vi "SET AO.vi"(8 "error in (no error)":errorcluster, 10 "Cluster SET AO":T1) -> (0 "error out":errorcluster)   [LabVIEW 2019]
uses:
  SET ARRAY AO.ctl
  SET SINGLE AO.ctl
  AO List.ctl
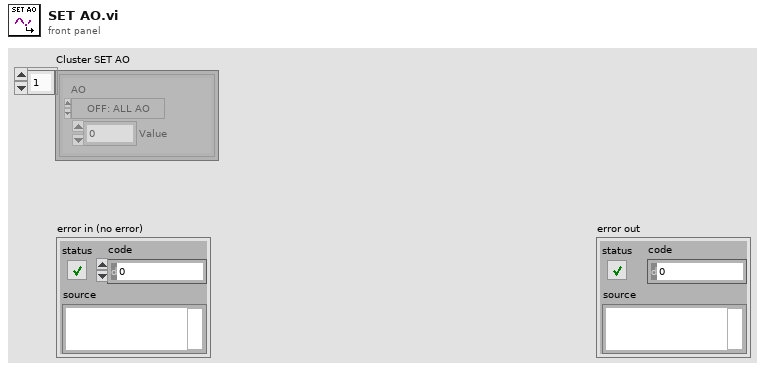
[diagram p1: front panel]
types:
  T1 = typedef "SET ARRAY AO.ctl" = T2[]
  T2 = typedef "SET SINGLE AO.ctl" = cluster{"AO":T3, "Value":dbl}
  T3 = typedef "AO List.ctl" = enum16{"OFF: ALL AO", "RIF VEL FRENO 1", "RIF VEL FRENO 2", "RIF VEL FRENO 3", "RIF COPPIA FRENO", "RIF COPPIA FRENO 1", "RIF COPPIA FRENO 2", "RIF COPPIA FRENO 3", "RIF CORRENTE FRENO 2", "RIF V ALIM 1", "RIF F ALIM 1", "RIF V ALIM 2", "RIF F ALIM 2", "RIF V ALIM 3", "RIF F ALIM 3", "RIF V ALIM 4", "RIF F ALIM 4", "FORZA AO PLC 3", "FORZA AO PLC 2", "FORZA AO PLC 1", "FORZA AO cDAQ", "Configura alimentatore keb", "Tempo rampa keb", "Condensatori", "Exit"}
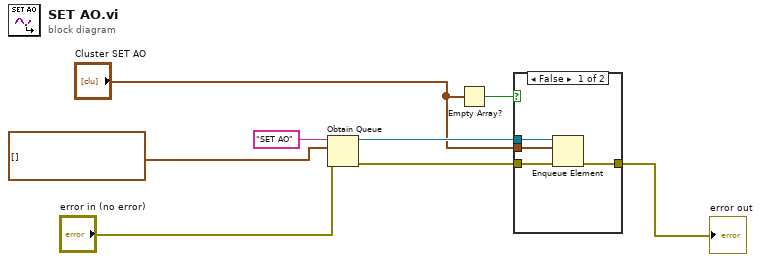
[diagram p0: block diagram]
diagram:
  n1 = Obtain Queue(name (unnamed)="SET AO", element data type=T1 [] ("Cluster SET AO"), error in (no error)="error in (no error)") -> (queue out=w7:refnum<queue>, error out=w6:errorcluster)  [unwired: 2 in, 1 out]
  n2 = Empty Array?(array="Cluster SET AO") -> (empty?=w1:bool)
  n3 = case shown="False" w1 {
    tunnel: w7 -> [w12 _]
    tunnel: w6 -> [w11 w13]
    tunnel: [w10 w13] -> w4
    tunnel: "Cluster SET AO" -> [w9 _]
    frame False {
      n4 = Enqueue Element(queue=w12, element=w9, error in (no error)=w11) -> (error out=w10:errorcluster)  [unwired: 1 in, 2 out]
    }
    frame True {
    }
  }
  "error out" <- w4
